vi "progress.vi"(10 "数值输入":i32, 11 "数值 3":i32) -> (2 "数值输出":dbl, 3 "字符串":string)   [LabVIEW 2018]
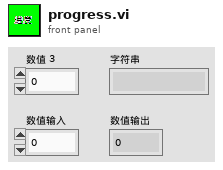
[diagram p1: front panel]
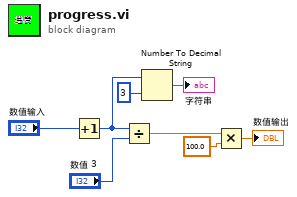
[diagram p0: block diagram]
diagram:
  n1 = Increment(x="数值输入") -> (x+1=w1:i32)
  n2 = Divide(x=w1, y="数值 3") -> (x/y=w4:dbl)
  n3 = Number To Decimal String(number=w1, width (-)=i16 3 ("宽度(-)")) -> (decimal integer string=→"字符串":string)
  n4 = Multiply(x=w4, y=100.0) -> (x*y=→"数值输出":dbl)
